vi "LED_I2C_clear.vi"(2 "Error In":errorcluster, 4 "Servo Controller Index":u8) -> (0 "Error Out":errorcluster)   [LabVIEW 2013]
uses:
  <vilib>/myRIO/Instrument Drivers/Onboard IO/I2C/vis/Smart Open.vi
  <vilib>/myRIO/Instrument Drivers/Onboard IO/I2C/vis/Configure.vi
  <vilib>/myRIO/Instrument Drivers/Onboard IO/I2C/vis/Write.vi
  <vilib>/myRIO/Instrument Drivers/Onboard IO/I2C/vis/Open.vi
  <vilib>/myRIO/Common/Instrument Driver Framework/myRIO v1.0/I2C/vis/myRIO v1.1 Open I2C.vi
  <vilib>/myRIO/Common/Instrument Driver Framework/Utilities/vis/Validate Channels.vi
  <vilib>/myRIO/Common/Instrument Driver Framework/myRIO v1.0/I2C/vis/myRIO v1.0 Reserve I2C.vi
  <vilib>/myRIO/Common/Instrument Driver Framework/myRIO v1.0/I2C/vis/myRIO v1.0 Build MUX Configuration I2C.vi
  <vilib>/myRIO/Common/Instrument Driver Framework/myRIO v1.0/Resource Manager/vis/myRIO v1.0 Reserve Channel List.vi
  <vilib>/myRIO/Common/Instrument Driver Framework/myRIO v1.0/Resource Manager/vis/myRIO v1.0 Create Configuration List.vi
  <vilib>/myRIO/Common/Instrument Driver Framework/myRIO v1.0/Resource Manager/vis/myRIO v1.0 Reserve Channel.vi
  <vilib>/myRIO/Common/Instrument Driver Framework/myRIO v1.0/Resource Manager/vis/myRIO v1.0 Unreserve Channel.vi
  <vilib>/myRIO/Common/Instrument Driver Framework/myRIO v1.0/Resource Manager/vis/myRIO v1.0 Build Mutex Name.vi
  <vilib>/myRIO/Common/Instrument Driver Framework/myRIO v1.0/myRIO v1.1 Open.vi
  <vilib>/Utility/VariantDataType/GetNumericInfo.vi
  <vilib>/Utility/error.llb/Error Cluster From Error Code.vi
  <vilib>/myRIO/Common/Instrument Driver Framework/Utilities/vis/IO Manager.vi
  <vilib>/myRIO/Common/Instrument Driver Framework/Utilities/vis/Configuration Manager.vi
  <vilib>/myRIO/Common/Instrument Driver Framework/myRIO v1.0/Resource Manager/vis/myRIO v1.0 Configure IO.vi
  <vilib>/myRIO/Common/Instrument Driver Framework/myRIO v1.0/myRIO v1.0 Close.vi
  <vilib>/myRIO/Common/Instrument Driver Framework/myRIO v1.0/I2C/vis/myRIO v1.0 Configure I2C.vi
  <vilib>/myRIO/Common/Instrument Driver Framework/myRIO v1.0/I2C/vis/myRIO v1.0 Write I2C.vi
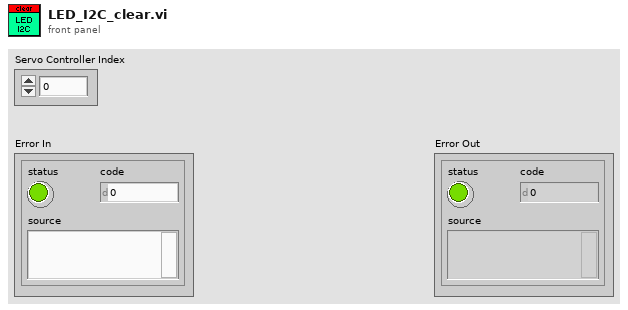
[diagram p1: front panel]
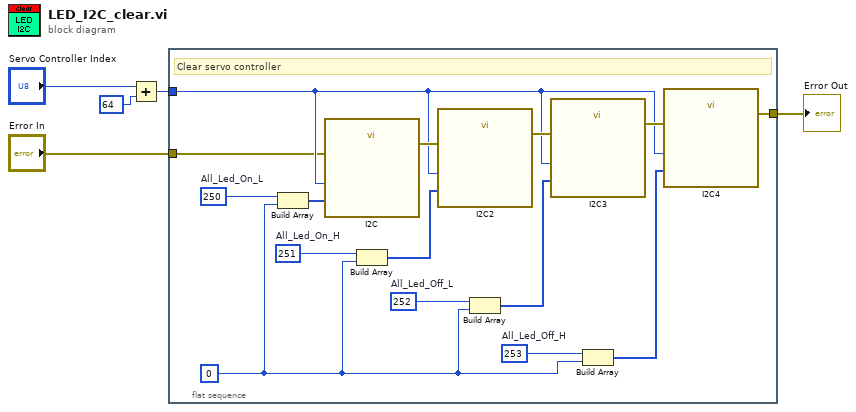
[diagram p0: block diagram]
diagram:
  n1 = Add(x="Servo Controller Index", y=u8 64 ("Slave Address (7-bit)")) -> (x+y=w4:u8)
  n2 = flat-sequence {
    tunnel: [w16] -> w3
    tunnel: w4 -> [w15]
    tunnel: "Error In" -> [w6]
    frame #0 {
      w11 = u8 253  # All_Led_Off_H
      w12 = u8 252  # All_Led_Off_L
      w13 = u8 251  # All_Led_On_H
      w7 = u8 0
      w14 = u8 250  # All_Led_On_L
      # "Clear servo controller"
      n3 = Build Array(w14, w7) -> (w20:u8[])
      n4 = call "I2C"("Slave Address (7-bit)"=w15, "Bytes to Write"=w20, "error in (no error)"=w6) -> ("error out"=w19:errorcluster)  [unwired: 24 in]
      n5 = Build Array(w13, w7) -> (w10:u8[])
      n6 = call "I2C2"("Slave Address (7-bit)"=w15, "Bytes to Write"=w10, "error in (no error)"=w19) -> ("error out"=w18:errorcluster)  [unwired: 24 in]
      n7 = Build Array(w12, w7) -> (w9:u8[])
      n8 = call "I2C3"("Slave Address (7-bit)"=w15, "Bytes to Write"=w9, "error in (no error)"=w18) -> ("error out"=w17:errorcluster)  [unwired: 24 in]
      n9 = Build Array(w11, w7) -> (w8:u8[])
      n10 = call "I2C4"("Slave Address (7-bit)"=w15, "Bytes to Write"=w8, "error in (no error)"=w17) -> ("error out"=w16:errorcluster)  [unwired: 24 in]
    }
  }
  "Error Out" <- w3
